vi "destroyAckCMDEvent.vi"(8 "error in (no error)":errorcluster, 11 "PubSubDataEvent in":refnum<class "PubSubDataEvent.lvclass">) -> (0 "error out":errorcluster, 3 "PubSubDataEvent out":refnum<class "PubSubDataEvent.lvclass">)   [LabVIEW 2016, in "PubSubDataEvent.lvclass"]
uses:
  PubSubDataEvent.lvclass
  PubSubDataEvent.lvclass/PubSubDataEvent.ctl
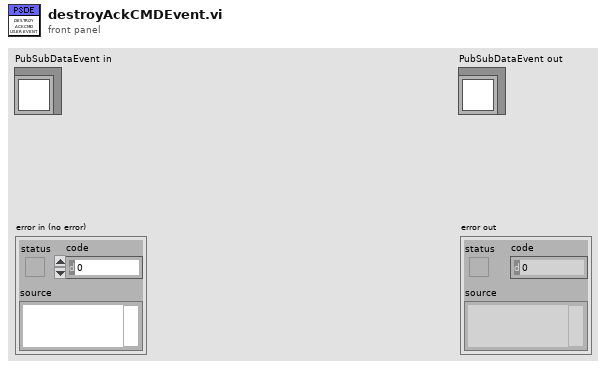
[diagram p1: front panel]
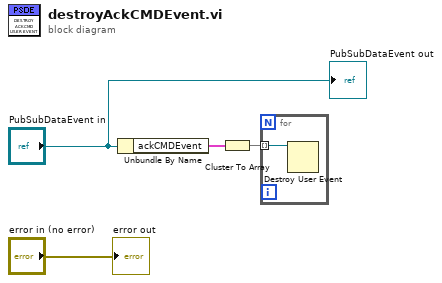
[diagram p0: block diagram]
diagram:
  n1 = Unbundle By Name("PubSubDataEvent in") -> ("ackCMDEvent"=w1:cluster{"ackCMD":refnum<user-event>})
  n2 = Cluster To Array(cluster=w1) -> (array=w2:refnum<user-event>[])
  n3 = for {
    tunnel: w2 -> [w5] mode=indexing
    n4 = Destroy User Event(user event=w5) -> ()  [unwired: 1 in, 1 out]
  }
  "error out" <- "error in (no error)"
  "PubSubDataEvent out" <- "PubSubDataEvent in"
